vi "Bucle Control T-RH-N2 +Log.vi"() -> ()   [LabVIEW 2015, in "VIPM2.lvlib"]
uses:
  VIPM2.lvlib
panel:
  in  "VISA resource name\nFlow valve":refnum<visa-resource-name>="COM3"
  out "time":dbl format="%#.2p"
  out "barra":i32(slide) scale=0.0..5.0
  out "Dew Point":string
  in  "Humidity setpoint":sgl=22.0 min=0 max=100 step=1 format="%#.2g%%RH"
  out "N2 flow (l/min)":sgl format="%#.3g"
  out "Flow-valve temperature":sgl format="%#.2g °C"
  out "Q N2 setpoint (l/min)":sgl format="%#_3g"
  out "Waveform Chart":T1(graph)
  out "error out":errorcluster
  out "Humidity String":string caption="Relative Humidity"
  out "Temperature String":string caption="Temperature"
  out "Sensor description":string
  in  "stop":bool
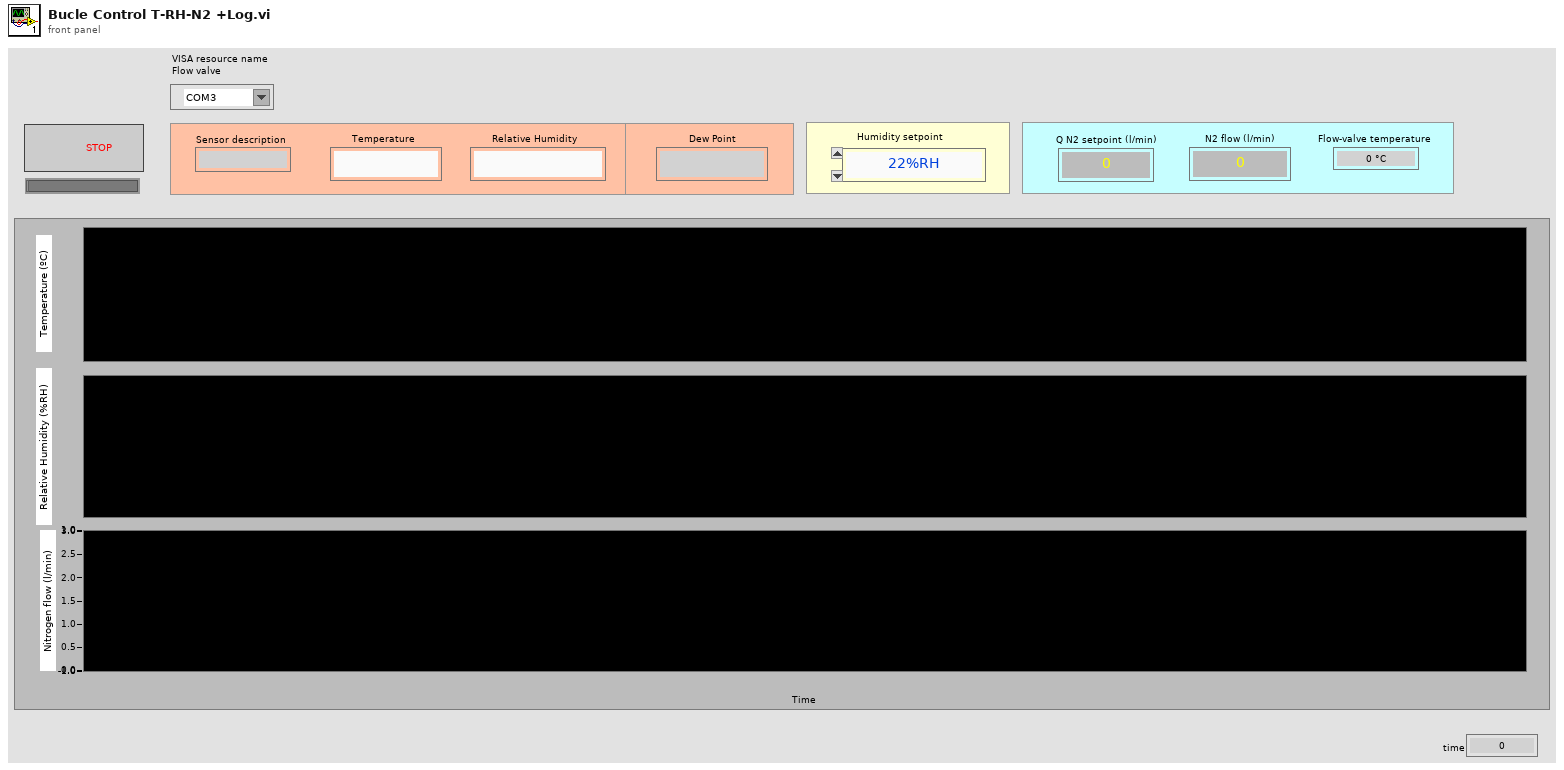
[diagram p1: front panel]
types:
  T1 = cluster{"Temperature":sgl, "Humidity":sgl, "Q N2 setpoint (l/min)":sgl}
  T2 = cluster{"Temperature":sgl, "Humidity":sgl, "Measure Direct":sgl}
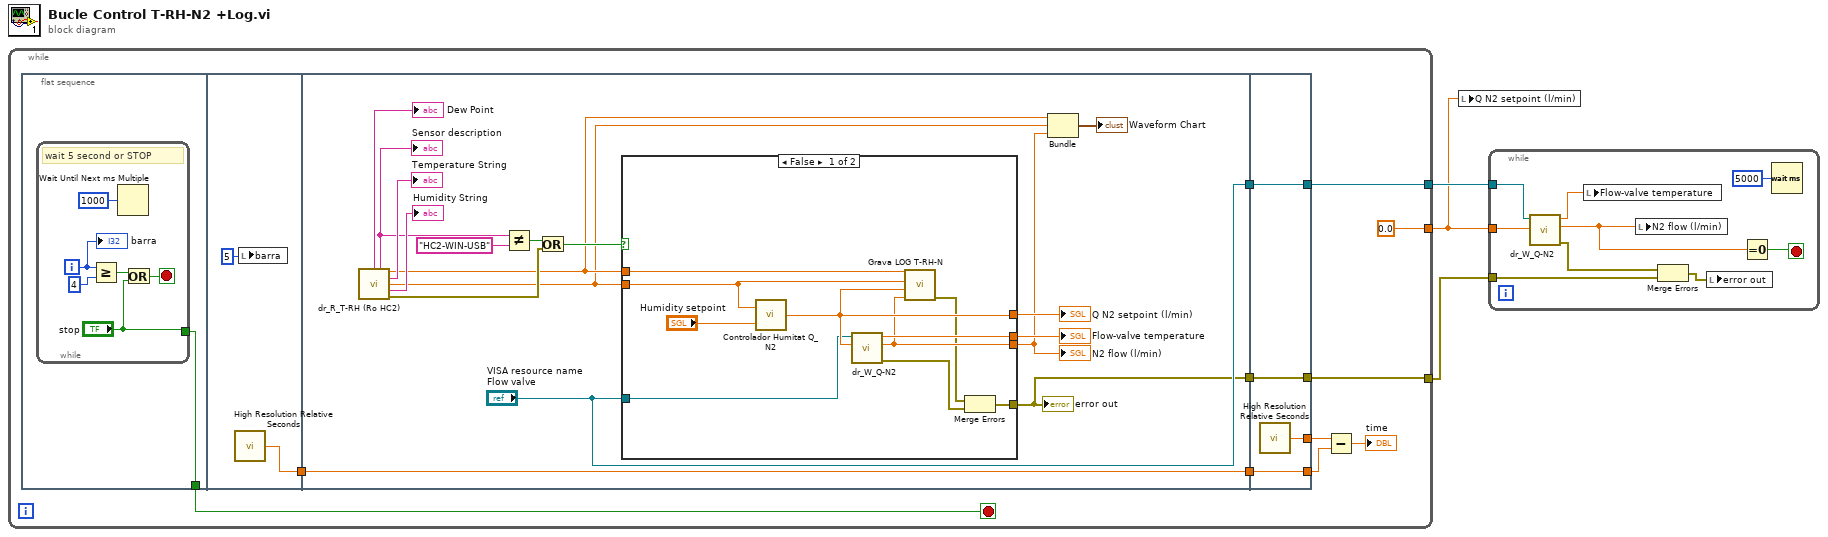
[diagram p0: block diagram]
diagram:
  n1 = while {
    tunnel: [sgl 0.0 ("Setpoint Direct")] -> w1
    tunnel: [w7] -> w3
    tunnel: [w4] -> w2
    stop <- w14 stop-if-true
    n2 = flat-sequence {
      tunnel: [w15] -> w14
      tunnel: [w22] -> w13
      tunnel: w13 -> [w26]
      tunnel: [w26] -> w12
      tunnel: ["VISA resource name\nFlow valve"] -> w6
      tunnel: [w24] -> w5
      tunnel: [w54] -> w11
      tunnel: [w53] -> w10
      tunnel: w12 -> [w53]
      tunnel: [w52] -> w7
      tunnel: w6 -> [w52]
      tunnel: [w51] -> w4
      tunnel: w5 -> [w51]
      frame #0 {
        n3 = while {
          tunnel: ["stop"] -> w15
          i -> [w16]
          stop <- w20 stop-if-true
          # "wait 5 second or STOP"
          n4 = Greater Or Equal?(x=w16, y=4) -> (x >= y?=w18:bool)
          n5 = Wait Until Next ms Multiple(millisecond multiple=u32 1000) -> ()  [unwired: 1 out]
          n6 = Or(x=w18, y="stop") -> (x .or. y?=w20:bool)
          "barra" <- w16
        }
      }
      frame #1 {
        n7 = call <vilib>:"High Resolution Relative Seconds.vi"() -> ("relative seconds"=w22:dbl)
        n8 = local write "barra"(5 ("barra")) -> ()
      }
      frame #2 {
        n9 = call "dr_R_T-RH (Ro HC2).vi"() -> ("Dew Point String"=→"Dew Point":string, "Device description"=w38:string, "Temperature"=w32:sgl, "Temperature String"=→"Temperature String":string, "Humidity"=w31:sgl, "Humidity String"=→"Humidity String":string, "error out"=w35:errorcluster)  [unwired: 9 in]
        "Sensor description" <- w38
        n10 = Not Equal?(x=w38, y="HC2-WIN-USB") -> (x != y?=w36:bool)
        n11 = Or(x=w36, y=w35) -> (x .or. y?=w34:bool)
        n12 = case shown="False" w34 {
          tunnel: w32 -> [w50 _]
          tunnel: w31 -> [w49 _]
          tunnel: [w47 _] -> w30
          tunnel: [w46 _] -> w29
          tunnel: [w45 _] -> w28
          tunnel: [w42 _] -> w24
          tunnel: "VISA resource name\nFlow valve" -> [w41 _]
          frame False {
            n13 = call "Controlador Humitat Q_N2.vi"("Humidity setpoint (%RH)"="Humidity setpoint", "Humidity (%RH)"=w49) -> ("Q N2 setpoint (l/min)"=w47:sgl)  [unwired: 1 in]
            n14 = call "dr_W_Q-N2.vi"("Setpoint Direct"=w47, "VISA resource name\nFlow valve"=w41) -> ("error out"=w43:errorcluster, "Measure Direct"=w45:sgl, "Flow-valve temperature"=w46:sgl)  [unwired: 6 in, 1 out]
            n15 = call "Grava LOG T-RH-N.vi"("N2 flow"=w45, "N2 setpoint"=w47, "Humidity"=w49, "Temperature"=w50) -> ("error out"=w44:errorcluster)  [unwired: 7 in]
            n16 = Merge Errors(w44, w43) -> (w42:errorcluster)
          }
          frame True {
            # "error or not the HC2 sensor"
          }
        }
        "Q N2 setpoint (l/min)" <- w30
        "Flow-valve temperature" <- w29
        "N2 flow (l/min)" <- w28
        "error out" <- w24
        n17 = Bundle("Temperature"=w32, "Humidity"=w31, "Measure Direct"=w28) -> (→"Waveform Chart":T2)  [unwired: 1 in]
      }
      frame #3 {
        n18 = call <vilib>:"High Resolution Relative Seconds.vi"() -> ("relative seconds"=w54:dbl)
      }
    }
    n19 = Subtract(x=w11, y=w10) -> (x-y=→"time":dbl)
  }
  n20 = local write "Q N2 setpoint (l/min)"(w1) -> ()
  n21 = while {
    tunnel: w1 -> [w63]
    tunnel: w3 -> [w58]
    tunnel: w2 -> [w56]
    stop <- w62 stop-if-true
    n22 = call "dr_W_Q-N2.vi"("Setpoint Direct"=w63, "VISA resource name\nFlow valve"=w58) -> ("error out"=w57:errorcluster, "Measure Direct"=w59:sgl, "Flow-valve temperature"=w60:sgl)  [unwired: 6 in, 1 out]
    n23 = local write "Flow-valve temperature"(w60) -> ()
    n24 = local write "N2 flow (l/min)"(w59) -> ()
    n25 = Merge Errors(w57, w56) -> (w55:errorcluster)
    n26 = local write "error out"(w55) -> ()
    n27 = Equal To 0?(x=w59) -> (x = 0?=w62:bool)
    n28 = Wait (ms)(milliseconds to wait=u32 5000) -> ()  [unwired: 1 out]
  }
